vi "Q -- get  number in range.vi"(4 "right":dbl=inf, 6 "left":dbl=-inf, 11 "fraction":dbl=11.0) -> (3 "number in range":dbl)   [LabVIEW 2015]
uses:
  Q - not nan -- real.vi
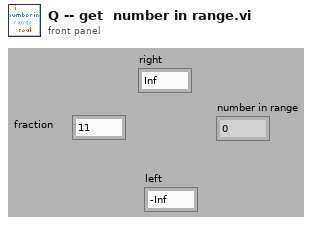
[diagram p1: front panel]
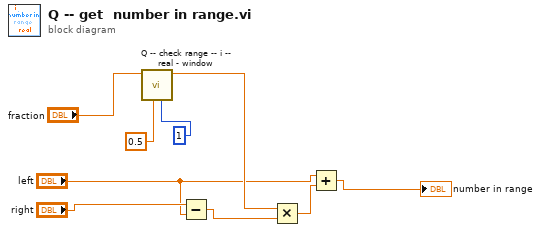
[diagram p0: block diagram]
diagram:
  n1 = call "Q -- check range -- i -- real - window.vi"("window"=1, "center"=0.5, "number"="fraction") -> ("number in range"=w4:dbl)  [unwired: 6 in, 2 out]
  n2 = Subtract(x="right", y="left") -> (x-y=w8:dbl)
  n3 = Multiply(x=w4, y=w8) -> (x*y=w2:dbl)
  n4 = Add(x="left", y=w2) -> (x+y=→"number in range":dbl)
